vi "GenOdorCalSeqMultiMix.vi"(9 "Base Dilution":dbl=0.1, 10 "Missaleneouns Parems":T3={"Ctr Odor Valve"=14, "Water Mix Valve"=12, "Total Odor Flow"=425.0, "Total Flow Setpoint"=531.25, "Control Pressure Channel"=1, "Mix Water Pressure Channel"=2}, 11 "Calibration Refs":T4={"Pressure Controller List"=[2, 2, 2, 3, 4], "Ratio List"=[0.9, 0.7, 0.6, 0.1, 0.1], "Valve List"=[12, 12, 12, 0, 8]}) -> (0 "newRatio":bool[](array[boolean])=[TRUE, TRUE, TRUE, FALSE], 3 "Cal Ref OUt":T1(array[cluster])=[{"Ratio"=0.6, "Valve"=8, "Pressure Channel"=4}, {"Ratio"=0.7, "Valve"=8, "Pressure Channel"=4}, {"Ratio"=0.9, "Valve"=0, "Pressure Channel"=3}, {"Ratio"=0.9, "Valve"=8, "Pressure Channel"=4}], 4 "A5Idx":bool[](array[boolean])=[TRUE, TRUE, FALSE, FALSE], 5 "Possible Water Mix Ratios":dbl[](array[numeric]))   [LabVIEW 2016]
uses:
  <vilib>/imath/engines/lvmath/Plug In/_Char/NIMS_CH_character datatype.ctl
  <vilib>/imath/engines/lvmath2/RunTimeEngine/VariableToken/Support/NIMS_Vector Boolean Index to I32 Index.vi
  <vilib>/imath/engines/lvmath2/RunTimeEngine/IndexRead/NIMS V(V).vi
  <instcachedir>/0/NIMS V(V)_298D9CB7BFEB42B8BC8D9C3C28AE8C70.lvgen/NIMS V(V)_298D9CB7BFEB42B8BC8D9C3C28AE8C70_001.vi
  <vilib>/imathl/engines/lvmath/Functions/Error Handling/Create Error.vi
  <instcachedir>/0/NIMS V(V)_298D9CB7BFEB42B8BC8D9C3C28AE8C70.lvgen/NIMS V(V)_298D9CB7BFEB42B8BC8D9C3C28AE8C70_002.vi
  <vilib>/imath/engines/lvmath2/RunTimeEngine/IndexReplace/NIMS V(V)=V.vi
  <instcachedir>/0/NIMS V(V)=V_BE8E060C6E1D4A13ABFD54A163A3AD30.lvgen/NIMS V(V)=V_BE8E060C6E1D4A13ABFD54A163A3AD30_000.vi
  <vilib>/imath/engines/lvmath2/RunTimeEngine/ErrorHandling/NIMS_Create Error From Enums.vi
  <vilib>/imath/engines/lvmath2/RunTimeEngine/BuiltInFunctions/findnz/NIMS_[1o]_findnz(GRowV).vi
  <instcachedir>/0/NIMS_[1o]_findnz(GRowV)_656056C849EF4762B1F0843BDDDEF2FF.lvgen/NIMS_[1o]_findnz(GRowV)_656056C849EF4762B1F0843BDDDEF2FF_000.vi
  <vilib>/imath/engines/lvmath/Plug In/_Char/NIMS_CH_Character RV to String.vi
  <vilib>/imath/engines/lvmath2/RunTimeEngine/BuiltInFunctions/length/NIMS_length(GV).vi
  <instcachedir>/0/NIMS_length(GV)_08A3D13377FD4E4B96F5795FBF3698FA.lvgen/NIMS_length(GV)_08A3D13377FD4E4B96F5795FBF3698FA_002.vi
  <vilib>/imath/engines/lvmath2/RunTimeEngine/BuiltInFunctions/random/NIMS_random.vi
  <vilib>/imath/engines/lvmath2/RunTimeSupport/NIMS_Error if Not Equal.vi
  <instcachedir>/0/NIMS_Error if Not Equal_EBDB539BFBF84063AF66BAE64AA6DE72.lvgen/NIMS_Error if Not Equal_EBDB539BFBF84063AF66BAE64AA6DE72_002.vi
  <vilib>/imath/engines/lvmath2/RunTimeEngine/IndexRead/NIMS V(M).vi
  <instcachedir>/0/NIMS V(M)_9C733378D59448EDB8B370EA0429D12A.lvgen/NIMS V(M)_9C733378D59448EDB8B370EA0429D12A_002.vi
  <instcachedir>/0/NIMS V(M)_9C733378D59448EDB8B370EA0429D12A.lvgen/NIMS V(M)_9C733378D59448EDB8B370EA0429D12A_001.vi
  <vilib>/imath/engines/lvmath2/RunTimeEngine/IndexReplace/NIMS V(V)=M.vi
  <instcachedir>/0/NIMS V(V)=M_4E1E70A83EF34EDC81D1F331EC25431D.lvgen/NIMS V(V)=M_4E1E70A83EF34EDC81D1F331EC25431D_001.vi
  <instcachedir>/0/NIMS V(M)_9C733378D59448EDB8B370EA0429D12A.lvgen/NIMS V(M)_9C733378D59448EDB8B370EA0429D12A_000.vi
  <instcachedir>/0/NIMS V(V)=M_4E1E70A83EF34EDC81D1F331EC25431D.lvgen/NIMS V(V)=M_4E1E70A83EF34EDC81D1F331EC25431D_002.vi
  <vilib>/imath/engines/lvmath2/RunTimeEngine/RowToken/NIMS_RowToken_CV_CV.vi
  <instcachedir>/0/NIMS_RowToken_CV_CV_29BB6DD8ABFD4F0A8989877FD0EDC468.lvgen/NIMS_RowToken_CV_CV_29BB6DD8ABFD4F0A8989877FD0EDC468_000.vi
  <vilib>/imath/engines/lvmath2/RunTimeEngine/BuiltInFunctions/sets_unique/NIMS_sets_unique(RM,Str).vi
  <instcachedir>/0/NIMS_sets_unique(RM,Str)_A8EF9DE225B84C3BB86CCEC66F55C59E.lvgen/NIMS_sets_unique(RM,Str)_A8EF9DE225B84C3BB86CCEC66F55C59E_001.vi
  <instcachedir>/0/NIMS V(V)_298D9CB7BFEB42B8BC8D9C3C28AE8C70.lvgen/NIMS V(V)_298D9CB7BFEB42B8BC8D9C3C28AE8C70_003.vi
  <instcachedir>/0/NIMS V(V)_298D9CB7BFEB42B8BC8D9C3C28AE8C70.lvgen/NIMS V(V)_298D9CB7BFEB42B8BC8D9C3C28AE8C70_000.vi
  <instcachedir>/0/NIMS_length(GV)_08A3D13377FD4E4B96F5795FBF3698FA.lvgen/NIMS_length(GV)_08A3D13377FD4E4B96F5795FBF3698FA_000.vi
  <vilib>/imath/engines/lvmath2/RunTimeEngine/RangeToken/NIMS_Range_R2 - Integer.vi
  <instcachedir>/0/NIMS_Range_R2 - Integer_416A044C4F024DBE8E97DA138CB3186F.lvgen/NIMS_Range_R2 - Integer_416A044C4F024DBE8E97DA138CB3186F_000.vi
  <vilib>/imath/engines/lvmath2/RunTimeEngine/CommandStatement/MC_CommandStatement_break.vi
  <vilib>/imath/engines/lvmath2/RunTimeEngine/IndexRead/NIMS V(S).vi
  <instcachedir>/0/NIMS V(S)_0488751826AF41519A22953C041130DC.lvgen/NIMS V(S)_0488751826AF41519A22953C041130DC_000.vi
  <vilib>/imath/engines/lvmath2/RunTimeEngine/IndexRead/NIMS V(R2).vi
  <instcachedir>/0/NIMS V(R2)_C76619605A0E4E9F8B2FA9389712AC47.lvgen/NIMS V(R2)_C76619605A0E4E9F8B2FA9389712AC47_000.vi
  <vilib>/imath/engines/lvmath2/RunTimeEngine/BuiltInFunctions/any/NIMS_any(GRowV).vi
  <vilib>/imath/engines/lvmath2/RunTimeEngine/IndexReplace/NIMS V(S)=V.vi
  <instcachedir>/0/NIMS V(S)=V_16451AC3E73743A5BCE8279D025B19B1.lvgen/NIMS V(S)=V_16451AC3E73743A5BCE8279D025B19B1_000.vi
  <vilib>/imath/engines/lvmath2/RunTimeEngine/NodeEndStatement/NIMS_NodeEndStatement_Output.vi
  <instcachedir>/0/NIMS_NodeEndStatement_Output_53EC0D466D134D7ABD903AC30B43404B.lvgen/NIMS_NodeEndStatement_Output_53EC0D466D134D7ABD903AC30B43404B_013.vi
  <instcachedir>/0/NIMS_NodeEndStatement_Output_53EC0D466D134D7ABD903AC30B43404B.lvgen/NIMS_NodeEndStatement_Output_53EC0D466D134D7ABD903AC30B43404B_012.vi
  <instcachedir>/0/NIMS_NodeEndStatement_Output_53EC0D466D134D7ABD903AC30B43404B.lvgen/NIMS_NodeEndStatement_Output_53EC0D466D134D7ABD903AC30B43404B_011.vi
  <instcachedir>/0/NIMS_NodeEndStatement_Output_53EC0D466D134D7ABD903AC30B43404B.lvgen/NIMS_NodeEndStatement_Output_53EC0D466D134D7ABD903AC30B43404B_005.vi
  <vilib>/imath/engines/lvmath2/RunTimeEngine/ErrorHandling/NIMS_Finalize Error.vi
panel:
  in  "Cluster":T2
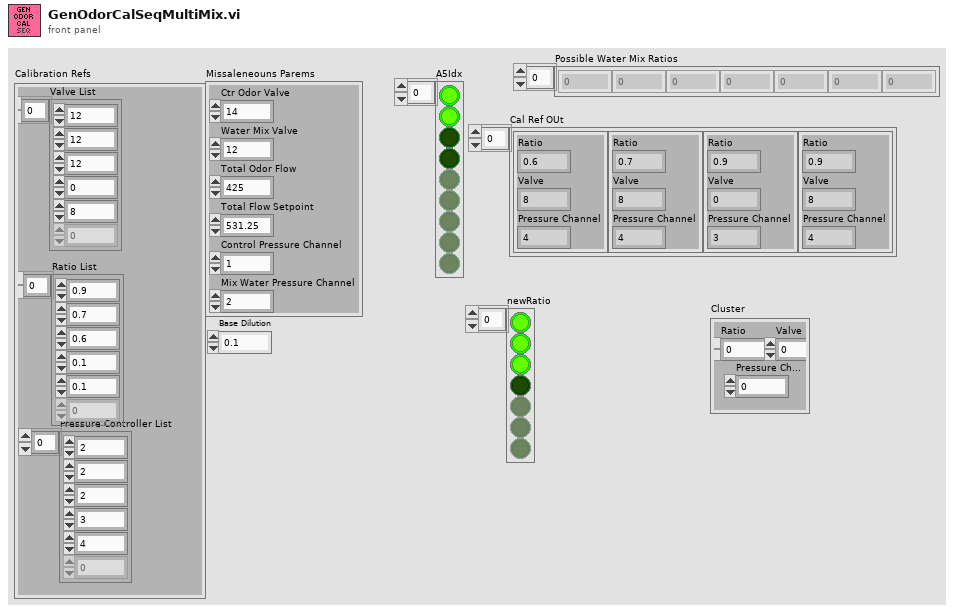
[diagram p1: front panel]
types:
  T1 = cluster{"Ratio":dbl, "Valve":u16, "Pressure Channel":u8}[]
  T2 = cluster{"Ratio":dbl, "Valve":u16, "Pressure Channel":u8}
  T3 = cluster{"Ctr Odor Valve":u16, "Water Mix Valve":u16, "Total Odor Flow":dbl, "Total Flow Setpoint":dbl, "Control Pressure Channel":u16, "Mix Water Pressure Channel":u16}
  T4 = cluster{"Pressure Controller List":u8[], "Ratio List":dbl[], "Valve List":u16[]}
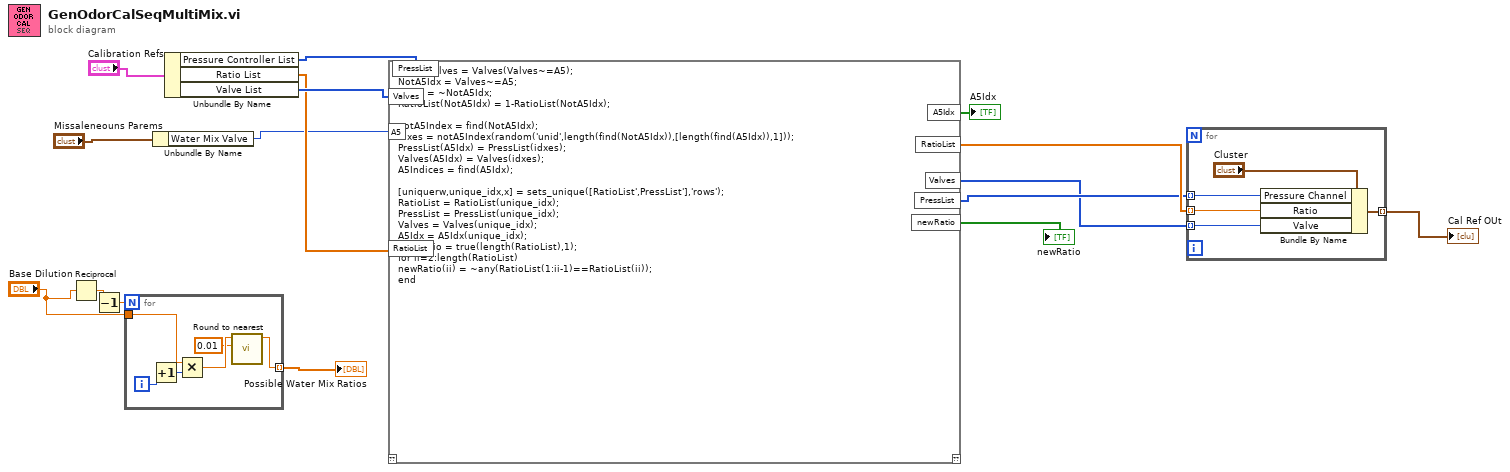
[diagram p0: block diagram]
diagram:
  n1 = Reciprocal(x="Base Dilution") -> (1/x=w14:dbl)
  n2 = Decrement(x=w14) -> (x-1=w8:dbl)
  n3 = for {
    N: w8 -> [_]
    tunnel: "Base Dilution" -> [w21]
    tunnel: [w17] -> w16 mode=indexing
    i -> [w22]
    n4 = Increment(x=w22) -> (x+1=w20:i32)
    n5 = Multiply(x=w21, y=w20) -> (x*y=w19:dbl)
    n6 = call "Round to nearest.vi"("Round to nearest"=0.01, "Number"=w19) -> ("Rounded"=w17:dbl)  [unwired: 9 in]
  }
  "Possible Water Mix Ratios" <- w16
  n7 = Unbundle By Name("Missaleneouns Parems") -> ("Water Mix Valve"=w9:u16)
  n8 = Unbundle By Name("Calibration Refs") -> ("Pressure Controller List"=w13:u8[], "Ratio List"=w11:dbl[], "Valve List"=w12:u16[])
  n9 = mathscript code="NotA5Valves = Valves(Valves~=A5);\nNotA5Idx = Valves~=A5;\nA5Idx = ~NotA5Idx;\nRatioList(NotA5Idx) = 1-RatioList(NotA5Idx);\n\nnotA5Index = find(NotA5Idx);\nidxes = notA5Index(random('unid',length(find(NotA5Idx)),[length(find(A5Idx)),1]));\nPressList(A5Idx) = PressList(idxes);\nValves(A5Idx) = Valves(idxes);\nA5Indices = find(A5Idx);\n\n[uniquerw,unique_idx,x] = sets_unique([RatioList',PressList'],'rows');\nRatioList = RatioList(unique_idx);\nPressList = PressList(unique_idx);\nValves = Valves(unique_idx);\nA5Idx = A5Idx(unique_idx);\nnewRatio = true(length(RatioList),1);\nfor ii=2:length(RatioList)\nnewRatio(ii) = ~any(RatioList(1:ii-1)==RatioList(ii));\nend"("A5"=w9, "Valves"=w12, "PressList"=w13, "RatioList"=w11) -> ("RatioList"=w5:dbl[], "Valves"=w3:u16[], "PressList"=w4:u8[], "A5Idx"=→"A5Idx":bool[], "newRatio"=→"newRatio":bool[])  [unwired: 1 in, 1 out]
  n10 = for {
    tunnel: w5 -> [w23] mode=indexing
    tunnel: w4 -> [w27] mode=indexing
    tunnel: w3 -> [w26] mode=indexing
    tunnel: [w25] -> w2 mode=indexing
    n11 = Bundle By Name(cluster="Cluster", "Pressure Channel"=w27, "Ratio"=w23, "Valve"=w26) -> (w25:T2)
  }
  "Cal Ref OUt" <- w2
